vi "CRYDAT-RES file array processor.vi"(10 "Entire file contents":string, 11 "Filepath":path) -> (0 "Canceled":bool, 3 "Array of flat Data or Results":string[](array[string]))   [LabVIEW 2013]
uses:
  CRYMainGlobal.vi
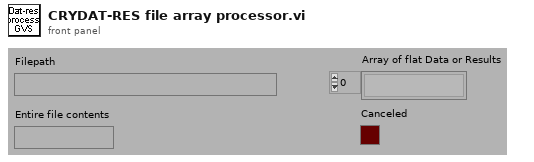
[diagram p1: front panel]
types:
  T1 = enum16{"OK", "Yes", "YesNo", "YesNoCancel", "ReplaceAppend"}
  T2 = typedef "CRYWaveform Cluster.ctl" = cluster{"Waveform":cluster{"X0":dbl, "dX":dbl, "Y":sgl[]}, "X data":u16, "Y data":u16, "Y axis":u16, "X unit":string, "Y unit":string, "Y dB ref":dbl, "display Y":bool, "display X":bool, "Overload?":bool, "Test Info":string, "Step No.":i32, "Name":string, "protected":bool, "Sqc history":string[], "Signal Channel ID":i32, "Plot Settings":cluster{"Color":u32, "Interpolation":u8, "Point Style":u8, "Line Style":u8, "Point Color":u32, "Line Width":u8, "Bar Plot Style":u8, "Fill To":i16}, "AutoProtect":bool}
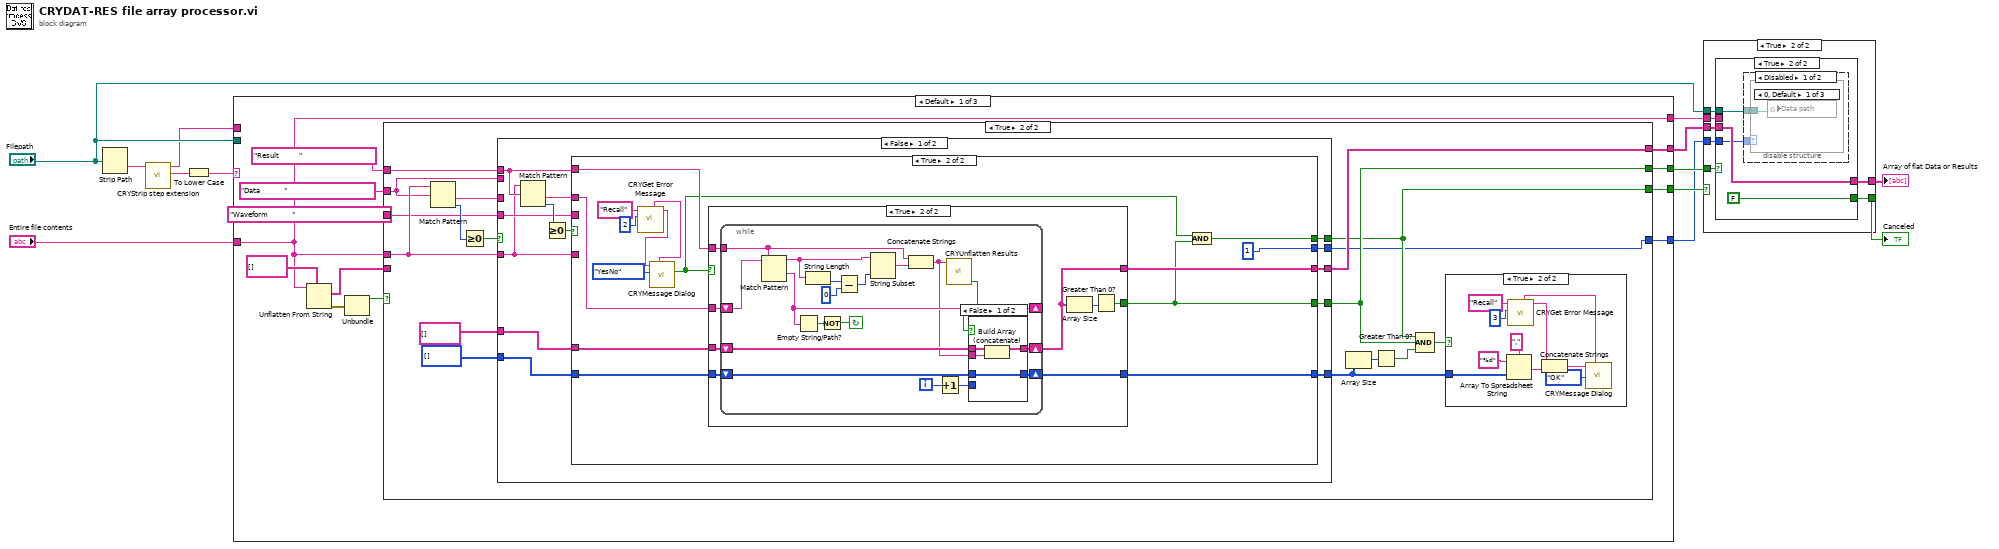
[diagram p0: block diagram]
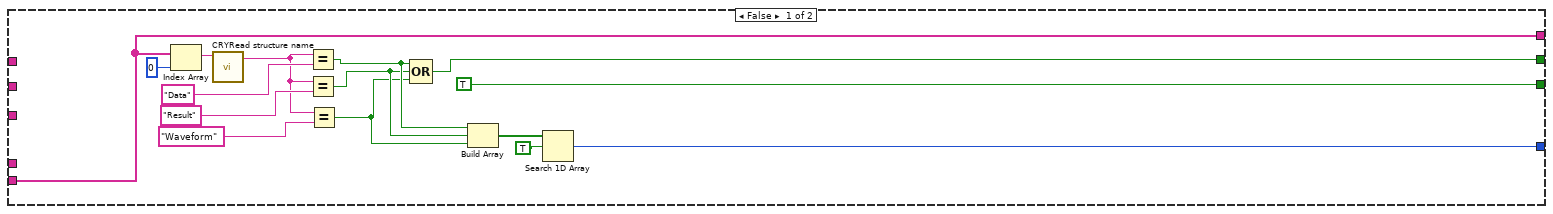
[diagram p2: hidden frame]
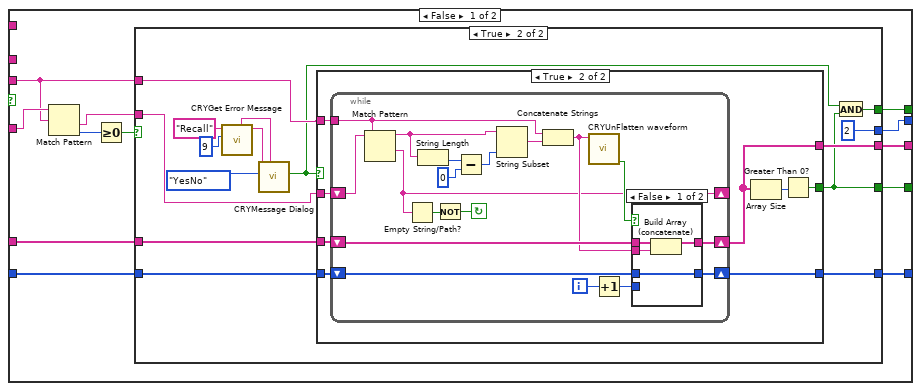
[diagram p4: hidden frame]
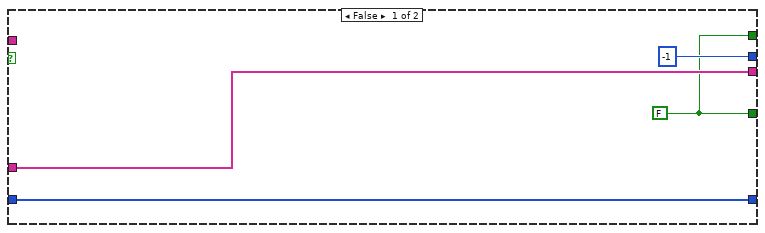
[diagram p5: hidden frame]
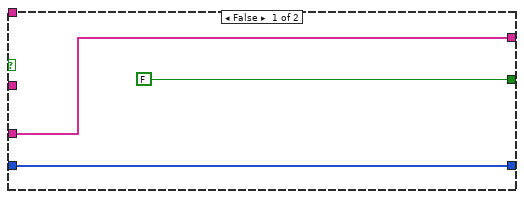
[diagram p6: hidden frame]
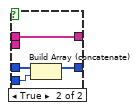
[diagram p7: hidden frame]
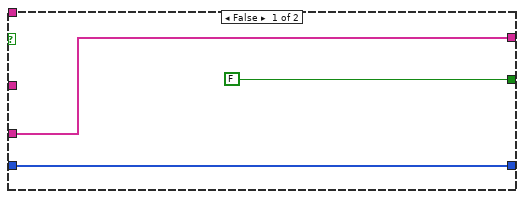
[diagram p8: hidden frame]
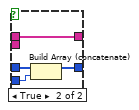
[diagram p9: hidden frame]
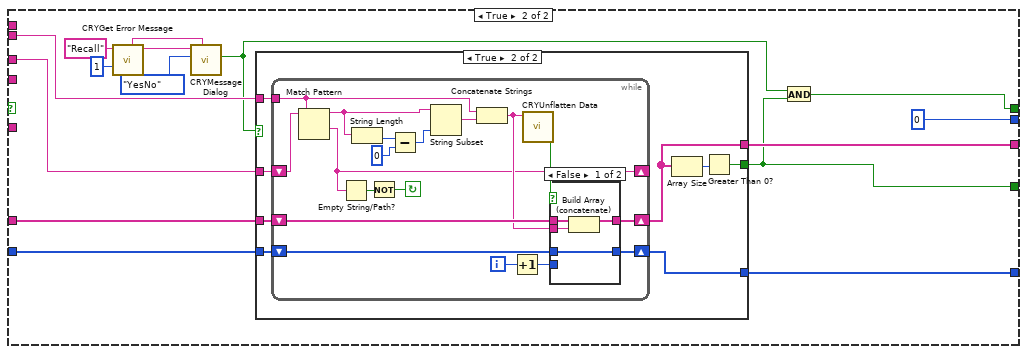
[diagram p10: hidden frame]
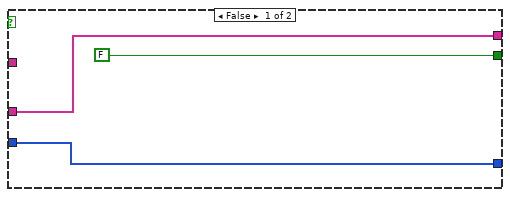
[diagram p11: hidden frame]
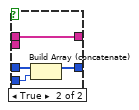
[diagram p12: hidden frame]
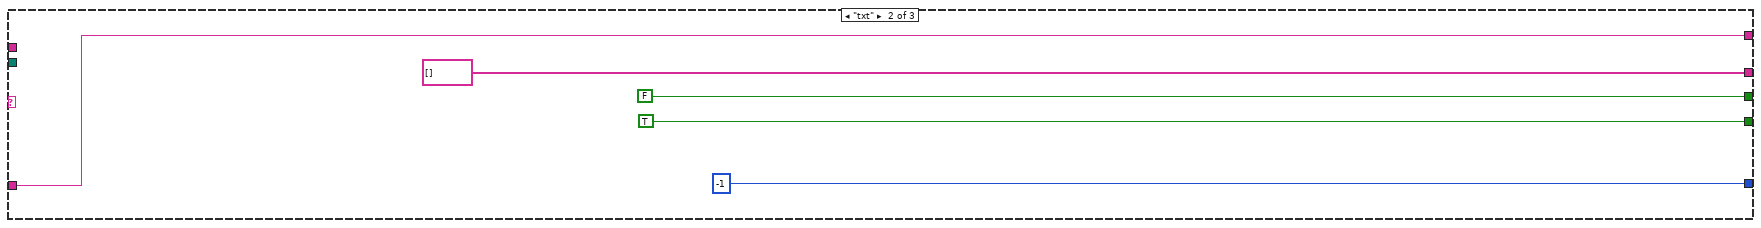
[diagram p13: hidden frame]
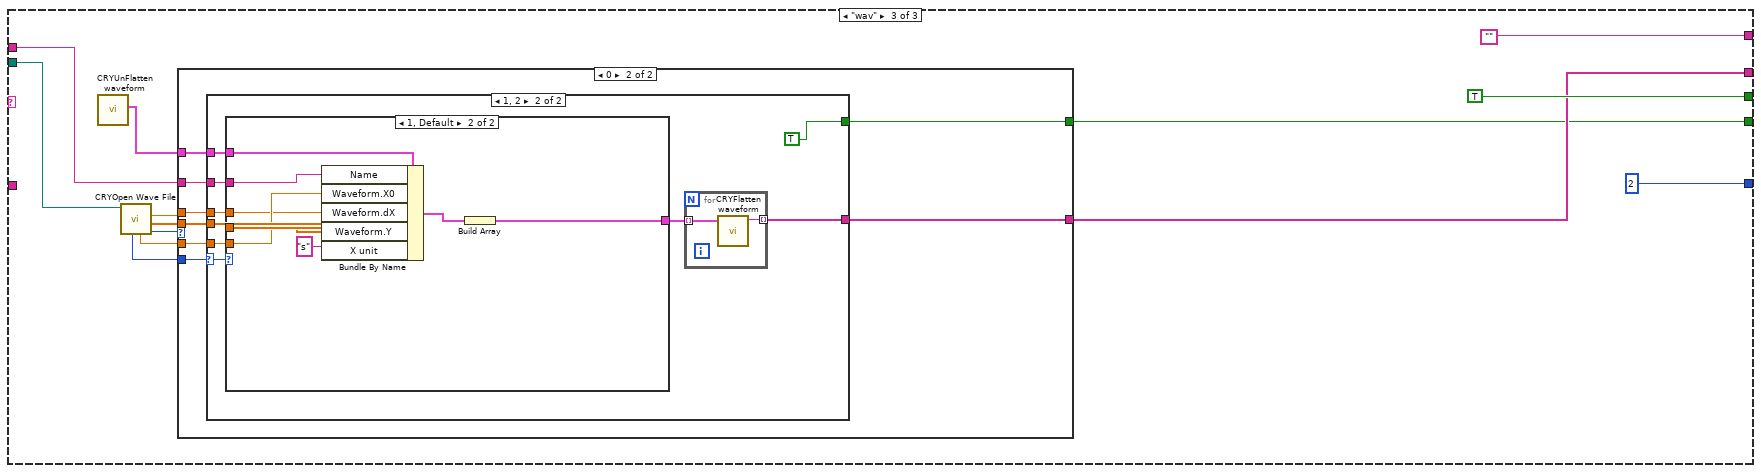
[diagram p14: hidden frame]
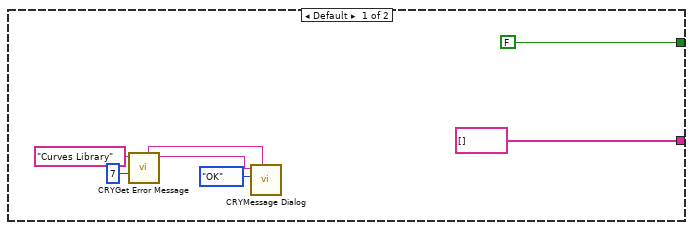
[diagram p15: hidden frame]
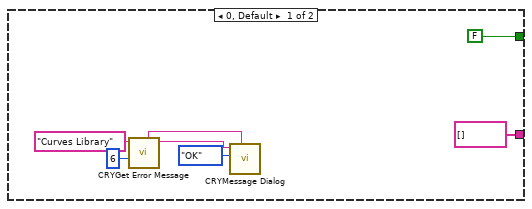
[diagram p16: hidden frame]
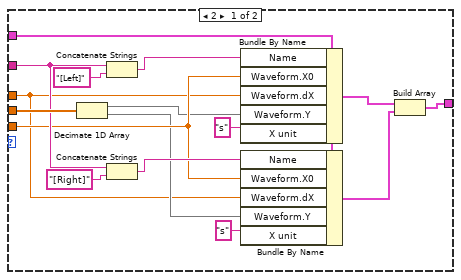
[diagram p17: hidden frame]
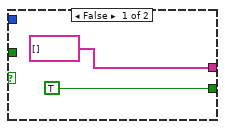
[diagram p18: hidden frame]
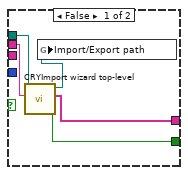
[diagram p19: hidden frame]
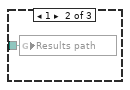
[diagram p20: hidden frame]
diagram:
  n1 = Strip Path(path="Filepath") -> (name=w7:string)  [unwired: 1 out]
  n2 = call "CRYStrip step extension.vi"("Step name w/ extension"=w7) -> ("Extension (3-letter category)"=w6:string, "Step name (base)"=w3:string)  [unwired: 7 in, 2 out]
  n3 = To Lower Case(string=w6) -> (all lower case string=w5:string)
  n4 = case shown="Default" w5 {
    tunnel: [w23 FALSE ("T button?") TRUE] -> w13
    tunnel: [w21 string[] [] w259] -> w10
    tunnel: [w18 w256 ""] -> w9
    tunnel: [w20 TRUE ("T button?") w258] -> w8
    tunnel: "Filepath" -> [_ _ w262]
    tunnel: w3 -> [_ _ w261]
    tunnel: "Entire file contents" -> [w18 w256 _]
    tunnel: [w14 -1 ("index of element") 2 ("index of element")] -> w1
    frame Default {
      n5 = Unflatten From String(type=string[] [], binary string=w18) -> (value=w22:string[], error out=w19:errorcluster)  [unwired: 1 in, 3 out]
      n6 = Unbundle(w19) -> ("status"=w24:bool)  [unwired: 2 out]
      n7 = case shown="True" w24 {
        tunnel: w22 -> [w35 _]
        tunnel: [w36 w48] -> w23
        tunnel: [w35 w53] -> w21
        tunnel: w18 -> [_ w54]
        tunnel: [TRUE ("T button?") w45] -> w20
        tunnel: "Result          " -> [_ w44]
        tunnel: "Data            " -> [_ w43]
        tunnel: "Waveform            " -> [_ w42]
        tunnel: [w26 w41] -> w14
        frame False {
          n8 = Index Array(array=w35, index=0 ("Index")) -> (element=w39:string)
          n9 = call "CRYRead structure name.vi"("Flat data structure"=w39) -> ("Data type"=w33:string)  [unwired: 7 in, 3 out]
          n10 = Equal?(x=w33, y="Data") -> (x = y?=w31:bool)
          n11 = Equal?(x=w33, y="Result") -> (x = y?=w30:bool)
          n12 = Equal?(x=w33, y="Waveform") -> (x = y?=w29:bool)
          n13 = Compound Arithmetic op=OR(w31, w30, w29) -> (w36:bool)
          n14 = Build Array(w31, w30, w29) -> (w28:bool[])
          n15 = Search 1D Array(1D array=w28, element=TRUE) -> (index of element=w26:i32)  [unwired: 1 in]
        }
        frame True {
          n16 = Match Pattern(string=w54, regular expression=w43) -> (after substring=w55:string, offset past match=w57:i32)  [unwired: 3 out]
          n17 = Greater Or Equal To 0?(x=w57) -> (x >= 0?=w56:bool)
          n18 = case shown="False" w56 {
            tunnel: w55 -> [_ w214]
            tunnel: w54 -> [w69 _]
            tunnel: w44 -> [w76 _]
            tunnel: [w78 w211] -> w53
            tunnel: w43 -> [_ w215]
            tunnel: string[] [] -> [w74 w213]
            tunnel: i32[] [] -> [w75 w212]
            tunnel: [w77 w202] -> w48
            tunnel: [w72 w210] -> w49
            tunnel: [w71 w201] -> w45
            tunnel: w42 -> [w70 _]
            tunnel: [w68 0 ("index of element")] -> w41
            frame False {
              n19 = Match Pattern(string=w69, regular expression=w76) -> (after substring=w73:string, offset past match=w80:i32)  [unwired: 3 out]
              n20 = Greater Or Equal To 0?(x=w80) -> (x >= 0?=w79:bool)
              n21 = case shown="True" w79 {
                tunnel: [w82 w162] -> w78
                tunnel: [w83 w156] -> w77
                tunnel: w76 -> [_ w163]
                tunnel: w75 -> [w86 w161]
                tunnel: w74 -> [w85 w160]
                tunnel: w73 -> [_ w159]
                tunnel: [w84 w158] -> w72
                tunnel: [w92 w157] -> w71
                tunnel: w70 -> [w87 _]
                tunnel: w69 -> [w91 _]
                tunnel: [w81 1 ("index of element")] -> w68
                frame False {
                  n22 = Match Pattern(string=w91, regular expression=w87) -> (after substring=w88:string, offset past match=w90:i32)  [unwired: 3 out]
                  n23 = Greater Or Equal To 0?(x=w90) -> (x >= 0?=w89:bool)
                  n24 = case shown="True" w89 {
                    tunnel: [w93 w100] -> w92
                    tunnel: w88 -> [_ w105]
                    tunnel: w87 -> [_ w106]
                    tunnel: w86 -> [w94 w103]
                    tunnel: w85 -> [w95 w104]
                    tunnel: [w94 w102] -> w84
                    tunnel: [w93 w99] -> w83
                    tunnel: [w95 w101] -> w82
                    tunnel: [-1 ("index of element") 2 ("index of element")] -> w81
                    frame False {
                      w93 = FALSE
                    }
                    frame True {
                      n25 = call "CRYGet Error Message.vi"("Error No"=9, "Kind"="Recall") -> ("Message"=w109:string, "Window Title"=w107:string)  [unwired: 4 in, 4 out]
                      n26 = call "CRYMessage Dialog.vi"("Window Title"=w107, "YesNoCancel"=T1."YesNo", "Message Content"=w109) -> ("YesNo"=w98:bool)  [unwired: 7 in, 1 out]
                      n27 = case shown="True" w98 {
                        tunnel: w106 -> [_ w122]
                        tunnel: [w114 w120] -> w101
                        tunnel: [FALSE w119] -> w99
                        tunnel: w103 -> [w113 w118]
                        tunnel: w104 -> [w114 w117]
                        tunnel: w105 -> [_ w116]
                        tunnel: [w113 w115] -> w102
                        frame False {
                        }
                        frame True {
                          n28 = while {
                            shift-left: w118 -> [w129]
                            shift-right: [w128] -> w115
                            shift-left: w117 -> [w132]
                            shift-right: [w130] -> w120
                            shift-left: w116 -> [w134]
                            shift-right: [w125] -> _
                            tunnel: w122 -> [w140]
                            i -> [w127]
                            stop <- w123 continue-if-true
                            n29 = Match Pattern(string=w134, regular expression=w140) -> (before substring=w137:string, after substring=w125:string)  [unwired: 3 out]
                            n30 = Empty String/Path?(string/path=w125) -> (empty?=w124:bool)
                            n31 = String Length(string=w137) -> (length=w139:i32)
                            n32 = Not(x=w124) -> (.not. x?=w123:bool)
                            n33 = Subtract(x=w139, y=0) -> (x-y=w136:i32)
                            n34 = String Subset(string=w137, length (rest)=w136) -> (substring=w135:string)  [unwired: 1 out]
                            n35 = Concatenate Strings(w140, w135) -> (w131:string)
                            n36 = call "CRYUnFlatten waveform.vi"("Unflatten Waveform"=w131) -> ("Error?"=w133:bool)  [unwired: 8 in, 2 out]
                            n37 = Increment(x=w127) -> (x+1=w126:i32)
                            n38 = case shown="False" w133 {
                              tunnel: w132 -> [w144 w148]
                              tunnel: w131 -> [w143 _]
                              tunnel: [w142 w148] -> w130
                              tunnel: w129 -> [w141 w147]
                              tunnel: [w141 w146] -> w128
                              tunnel: w126 -> [_ w145]
                              frame False {
                                n39 = Build Array (concatenate)(w144, w143) -> (w142:string[])
                              }
                              frame True {
                                n40 = Build Array (concatenate)(w147, w145) -> (w146:i32[])
                              }
                            }
                          }
                          n41 = Array Size(array=w120) -> (size(s)=w121:i32)
                          n42 = Greater Than 0?(x=w121) -> (x > 0?=w119:bool)
                        }
                      }
                      n43 = And(x=w98, y=w99) -> (x .and. y?=w100:bool)
                    }
                  }
                }
                frame True {
                  n44 = call "CRYGet Error Message.vi"("Error No"=2, "Kind"="Recall") -> ("Message"=w153:string, "Window Title"=w150:string)  [unwired: 4 in, 4 out]
                  n45 = call "CRYMessage Dialog.vi"("Window Title"=w150, "YesNoCancel"=T1."YesNo", "Message Content"=w153) -> ("YesNo"=w151:bool)  [unwired: 7 in, 1 out]
                  n46 = case shown="True" w151 {
                    tunnel: w163 -> [_ w174]
                    tunnel: [w166 w172] -> w162
                    tunnel: [FALSE w171] -> w156
                    tunnel: w161 -> [w165 w170]
                    tunnel: w160 -> [w166 w169]
                    tunnel: w159 -> [_ w168]
                    tunnel: [w165 w167] -> w158
                    frame False {
                    }
                    frame True {
                      n47 = while {
                        shift-left: w170 -> [w183]
                        shift-right: [w182] -> w167
                        shift-left: w169 -> [w185]
                        shift-right: [w184] -> w172
                        shift-left: w168 -> [w186]
                        shift-right: [w180] -> _
                        tunnel: w174 -> [w192]
                        i -> [w181]
                        stop <- w178 continue-if-true
                        n48 = Match Pattern(string=w186, regular expression=w192) -> (before substring=w189:string, after substring=w180:string)  [unwired: 3 out]
                        n49 = Empty String/Path?(string/path=w180) -> (empty?=w179:bool)
                        n50 = String Length(string=w189) -> (length=w191:i32)
                        n51 = Not(x=w179) -> (.not. x?=w178:bool)
                        n52 = Subtract(x=w191, y=0) -> (x-y=w188:i32)
                        n53 = String Subset(string=w189, length (rest)=w188) -> (substring=w187:string)  [unwired: 1 out]
                        n54 = Concatenate Strings(w192, w187) -> (w175:string)
                        n55 = Increment(x=w181) -> (x+1=w177:i32)
                        n56 = call "CRYUnflatten Results.vi"("Unflatten Result"=w175) -> ("Error?"=w176:bool)  [unwired: 8 in, 2 out]
                        n57 = case shown="False" w176 {
                          tunnel: w185 -> [w196 w200]
                          tunnel: w175 -> [w195 _]
                          tunnel: [w194 w200] -> w184
                          tunnel: w183 -> [w193 w199]
                          tunnel: [w193 w198] -> w182
                          tunnel: w177 -> [_ w197]
                          frame False {
                            n58 = Build Array (concatenate)(w196, w195) -> (w194:string[])
                          }
                          frame True {
                            n59 = Build Array (concatenate)(w199, w197) -> (w198:i32[])
                          }
                        }
                      }
                      n60 = Array Size(array=w172) -> (size(s)=w173:i32)
                      n61 = Greater Than 0?(x=w173) -> (x > 0?=w171:bool)
                    }
                  }
                  n62 = And(x=w151, y=w156) -> (x .and. y?=w157:bool)
                }
              }
            }
            frame True {
              n63 = call "CRYGet Error Message.vi"("Error No"=1, "Kind"="Recall") -> ("Message"=w207:string, "Window Title"=w206:string)  [unwired: 4 in, 4 out]
              n64 = call "CRYMessage Dialog.vi"("Window Title"=w206, "YesNoCancel"=T1."YesNo", "Message Content"=w207) -> ("YesNo"=w203:bool)  [unwired: 7 in, 1 out]
              n65 = case shown="True" w203 {
                tunnel: w215 -> [_ w226]
                tunnel: w214 -> [_ w225]
                tunnel: w213 -> [w218 w224]
                tunnel: w212 -> [w217 w223]
                tunnel: [w218 w222] -> w211
                tunnel: [FALSE w220] -> w202
                tunnel: [w217 w219] -> w210
                frame False {
                }
                frame True {
                  n66 = while {
                    shift-left: w223 -> [w233]
                    shift-right: [w232] -> w219
                    shift-left: w224 -> [w236]
                    shift-right: [w234] -> w222
                    shift-left: w225 -> [w238]
                    shift-right: [w229] -> _
                    tunnel: w226 -> [w244]
                    i -> [w231]
                    stop <- w227 continue-if-true
                    n67 = Match Pattern(string=w238, regular expression=w244) -> (before substring=w241:string, after substring=w229:string)  [unwired: 3 out]
                    n68 = Empty String/Path?(string/path=w229) -> (empty?=w228:bool)
                    n69 = String Length(string=w241) -> (length=w243:i32)
                    n70 = Not(x=w228) -> (.not. x?=w227:bool)
                    n71 = Subtract(x=w243, y=0) -> (x-y=w240:i32)
                    n72 = String Subset(string=w241, length (rest)=w240) -> (substring=w239:string)  [unwired: 1 out]
                    n73 = Concatenate Strings(w244, w239) -> (w235:string)
                    n74 = Increment(x=w231) -> (x+1=w230:i32)
                    n75 = call "CRYUnflatten Data.vi"("Unflatten data"=w235) -> ("Error?"=w237:bool)  [unwired: 8 in, 2 out]
                    n76 = case shown="False" w237 {
                      tunnel: w236 -> [w248 w252]
                      tunnel: w235 -> [w247 _]
                      tunnel: [w246 w252] -> w234
                      tunnel: w233 -> [w245 w251]
                      tunnel: [w245 w250] -> w232
                      tunnel: w230 -> [_ w249]
                      frame False {
                        n77 = Build Array (concatenate)(w248, w247) -> (w246:string[])
                      }
                      frame True {
                        n78 = Build Array (concatenate)(w251, w249) -> (w250:i32[])
                      }
                    }
                  }
                  n79 = Array Size(array=w222) -> (size(s)=w221:i32)
                  n80 = Greater Than 0?(x=w221) -> (x > 0?=w220:bool)
                }
              }
              n81 = And(x=w203, y=w202) -> (x .and. y?=w201:bool)
            }
          }
          n82 = Array Size(array=w49) -> (size(s)=w50:i32)
          n83 = Greater Than 0?(x=w50) -> (x > 0?=w47:bool)
          n84 = Compound Arithmetic op=AND(w45, w48, w47) -> (w46:bool)
          n85 = case shown="True" w46 {
            tunnel: w49 -> [_ w64]
            frame False {
            }
            frame True {
              n86 = Array To Spreadsheet String(delimiter (Tab)=",", array=w64, 3:"%d" ("format string")) -> (spreadsheet string=w67:string)
              n87 = call "CRYGet Error Message.vi"("Error No"=3, "Kind"="Recall") -> ("Message"=w61:string, "Window Title"=w58:string)  [unwired: 4 in, 4 out]
              n88 = Concatenate Strings(w61, w67) -> (w60:string)
              n89 = call "CRYMessage Dialog.vi"("Window Title"=w58, "YesNoCancel"=T1."OK", "Message Content"=w60) -> ()  [unwired: 7 in, 2 out]
            }
          }
        }
      }
    }
    frame "txt" {
    }
    frame "wav" {
      n90 = call "CRYUnFlatten waveform.vi"() -> ("Waveform Cluster"=w260:T2)  [unwired: 9 in, 2 out]
      n91 = call "CRYOpen Wave File.vi"("Wave File Path In"=w262) -> ("Error Out(0-OK)"=w263:u32, "Wave Data Out"=w266:sgl[], "dT"=w265:dbl, "X0"=w264:dbl, "Channels"=w267:u32)  [unwired: 5 in, 1 out]
      n92 = case shown="0" w263 {
        tunnel: w260 -> [_ w285]
        tunnel: w264 -> [_ w284]
        tunnel: w265 -> [_ w283]
        tunnel: w266 -> [_ w282]
        tunnel: w267 -> [_ w281]
        tunnel: w261 -> [_ w280]
        tunnel: [string[] [] w279] -> w259
        tunnel: [FALSE w278] -> w258
        frame Default {
          n93 = call "CRYGet Error Message.vi"("Error No"=7, "Kind"="Curves Library") -> ("Message"=w273:string, "Window Title"=w274:string)  [unwired: 4 in, 4 out]
          n94 = call "CRYMessage Dialog.vi"("Window Title"=w274, "YesNoCancel"=T1."OK", "Message Content"=w273) -> ()  [unwired: 7 in, 2 out]
        }
        frame 0 {
          n95 = case shown="1, 2" w281 {
            selector: w281 -> [_ w297]
            tunnel: w285 -> [_ w301]
            tunnel: w284 -> [_ w300]
            tunnel: w283 -> [_ w299]
            tunnel: w282 -> [_ w298]
            tunnel: w280 -> [_ w296]
            tunnel: [string[] [] w294] -> w279
            tunnel: [FALSE TRUE] -> w278
            frame 0, Default {
              n96 = call "CRYGet Error Message.vi"("Error No"=6, "Kind"="Curves Library") -> ("Message"=w288:string, "Window Title"=w289:string)  [unwired: 4 in, 4 out]
              n97 = call "CRYMessage Dialog.vi"("Window Title"=w289, "YesNoCancel"=T1."OK", "Message Content"=w288) -> ()  [unwired: 7 in, 2 out]
            }
            frame 1, 2 {
              n98 = case shown="1, Default" w297 {
                tunnel: w301 -> [w312 w327]
                tunnel: w296 -> [w311 w324]
                tunnel: w300 -> [w310 w323]
                tunnel: w299 -> [w307 w322]
                tunnel: w298 -> [w318 w321]
                tunnel: [w304 w320] -> w295
                frame 2 {
                  n99 = Decimate 1D Array(w318) -> (w309:sgl[], w308:sgl[])
                  n100 = Concatenate Strings(w311, "[Left]" ("string")) -> (w316:string)
                  n101 = Concatenate Strings(w311, "[Right]" ("string")) -> (w315:string)
                  n102 = Bundle By Name(cluster=w312, "Name"=w316, "Waveform.X0"=w310, "Waveform.dX"=w307, "Waveform.Y"=w309, "X unit"="s") -> (w306:T2)
                  n103 = Bundle By Name(cluster=w312, "Name"=w315, "Waveform.X0"=w310, "Waveform.dX"=w307, "Waveform.Y"=w308, "X unit"="s") -> (w305:T2)
                  n104 = Build Array(w306, w305) -> (w304:T2[])
                }
                frame 1, Default {
                  n105 = Bundle By Name(cluster=w327, "Name"=w324, "Waveform.X0"=w323, "Waveform.dX"=w322, "Waveform.Y"=w321, "X unit"="s") -> (w326:T2)
                  n106 = Build Array(w326) -> (w320:T2[])
                }
              }
              n107 = for {
                tunnel: w295 -> [w303] mode=indexing
                tunnel: [w302] -> w294 mode=indexing
                n108 = call "CRYFlatten waveform.vi"("Waveform Cluster"=w303) -> ("Flatten Waveform"=w302:string)  [unwired: 10 in]
              }
            }
          }
        }
      }
    }
  }
  n109 = case shown="True" w8 {
    tunnel: w13 -> [_ w336]
    tunnel: "Filepath" -> [_ w335]
    tunnel: w1 -> [_ w334]
    tunnel: [TRUE ("Canceled?") w333] -> w12
    tunnel: [string[] [] ("Data array out") w332] -> w11
    tunnel: w10 -> [_ w331]
    tunnel: w9 -> [_ w330]
    frame False {
    }
    frame True {
      n110 = case shown="True" w336 {
        tunnel: w331 -> [_ w345]
        tunnel: [w341 w345] -> w332
        tunnel: [w340 FALSE ("Canceled?")] -> w333
        tunnel: w335 -> [w339 w343]
        tunnel: w330 -> [w338 _]
        tunnel: w334 -> [_ w342]
        frame False {
          n111 = call "CRYImport wizard top-level.vi"("Data in flat (default empty)"=w338, "Import path (just directory if no data input)"=w339) -> ("Canceled?"=w340:bool, "Data array out"=w341:string[], "Path out"=w337:path)  [unwired: 7 in]
          n112 = global write "CRYMainGlobal.vi" "Import/Export path"(w337) -> ()
        }
        frame True {
          n113 = disable-structure shown="Disabled" {
            disable-tunnel: w343 -> [w347 _]
            disable-tunnel: w342 -> [w346 _]
            frame Disabled {
              n114 = case shown="0, Default" w346 {
                tunnel: w347 -> [w348 w349 w350]
                frame 0, Default {
                  n115 = global write "CRYMainGlobal.vi" "Data path"(w348) -> ()
                }
                frame 1 {
                  n116 = global write "CRYMainGlobal.vi" "Results path"(w349) -> ()
                }
                frame 2 {
                  n117 = global write "CRYMainGlobal.vi" "Wave path"(w350) -> ()
                }
              }
            }
            frame Enabled {
            }
          }
        }
      }
    }
  }
  "Array of flat Data or Results" <- w11
  "Canceled" <- w12
